vi "WSVCAP SHL Host LL Manage FPGA Top Level Controls.vi"(0 "Value In":variant, 1 "FPGA VI Reference (Init Only)":refnum<k20>, 7 "FPGA Top Level Control":T1=enum."Read Status Flag", 11 "error in (no error)":errorcluster, 12 "Simulate FPGA (Init Only)":bool=TRUE, 13 "Operation":T2) -> (4 "Value Out":variant, 15 "error out":errorcluster)   [LabVIEW 2012]
uses:
  Type Defs/WSVCAP SHL Top Level Control Operation Enum.ctl
  Type Defs/WSVCAP SHL Top Level Control Enum.ctl
  Type Defs/WSVCAP SHL State.ctl
  Type Defs/WSVCAP SHL Transaction Enum.ctl
  <vilib>/Utility/error.llb/Error Cluster From Error Code.vi
  <vilib>/rvi/errors/niLvFpgaAdjustHostInterfaceError.vi
  <vilib>/rvi/interface/nirviReadWriteControl/nirviReadWriteControl.xnode
  FPGA Bitfiles/WSVCAPShell_WiSpryFPGA1_WSVCAPSHLFPGATLT_T3ca54mRgtw.lvbitx
  NiFpgaLv.dll
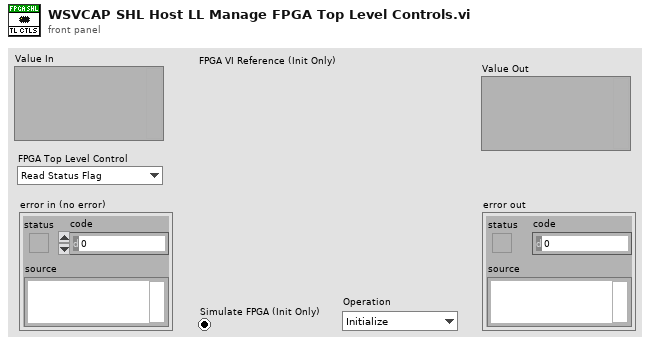
[diagram p1: front panel]
types:
  T1 = typedef "WSVCAP SHL Top Level Control Enum.ctl" = enum16{"Start", "Cmd", "Transaction", "Wait Ticks", "Socket Mask", "Slave Address", "Sub Address", "Bytes to Write", "Bytes to Read", "Write Data", "Write Flag", "Read Data", "Read Flag", "Ack Read", "Read Status Flag", "Ack Read Status", "Status", "Cycle Count", "Stop Cycle", "Exit"}
  T2 = typedef "WSVCAP SHL Top Level Control Operation Enum.ctl" = enum16{"Initialize", "Set Control", "Read Control", "Close"}
  T3 = typedef "WSVCAP SHL State.ctl" = enum8{"Idle", "Transfer Data"}
  T4 = typedef "WSVCAP SHL Transaction Enum.ctl" = enum16{"I2C-Read Data", "I2C-Write Data", "SPI-Write/Read Data", "RFFE-Ext Write", "RFFE-Ext Read"}
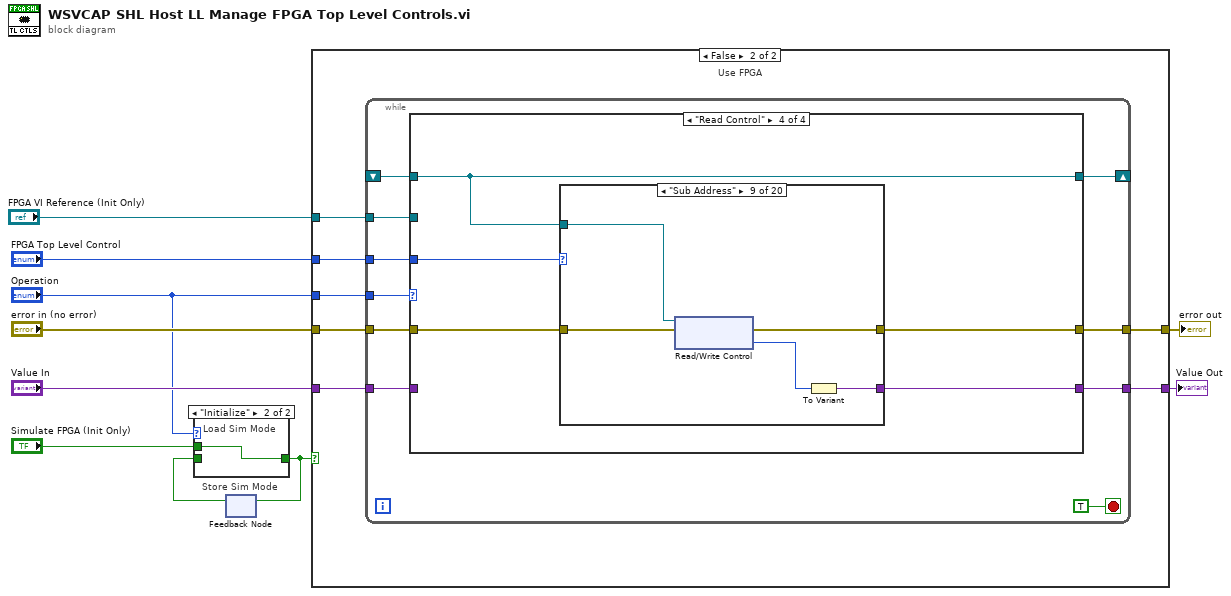
[diagram p0: block diagram]
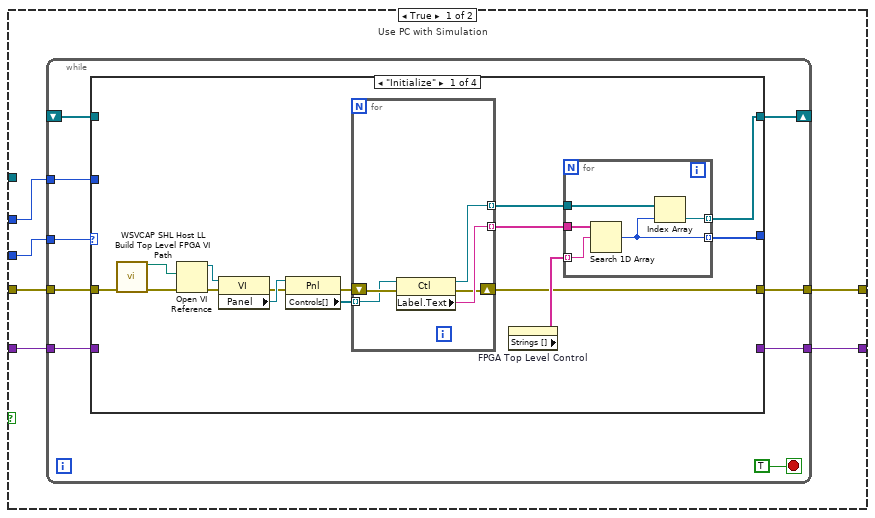
[diagram p2: hidden frame]
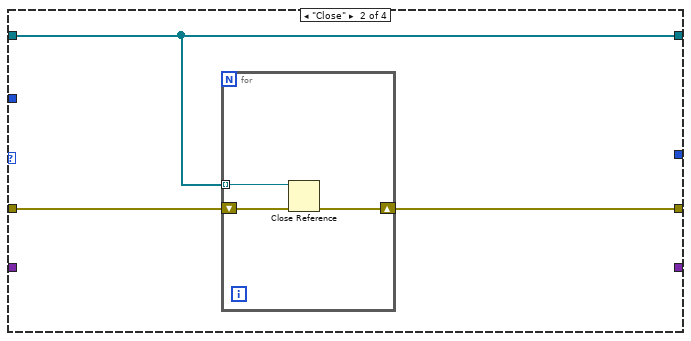
[diagram p3: hidden frame]
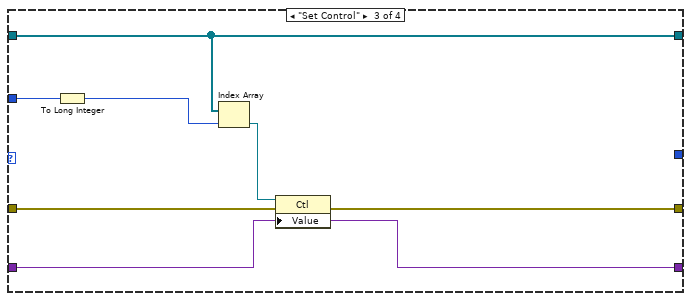
[diagram p4: hidden frame]
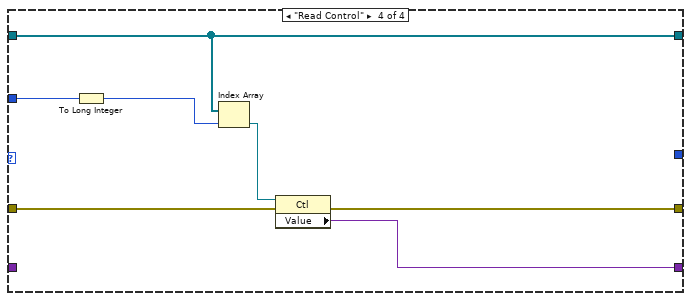
[diagram p5: hidden frame]
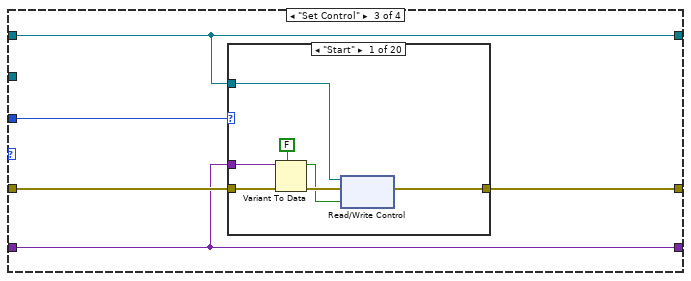
[diagram p8: hidden frame]
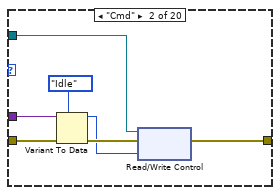
[diagram p9: hidden frame]
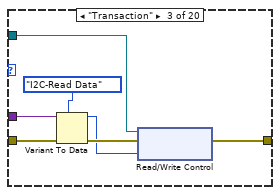
[diagram p10: hidden frame]
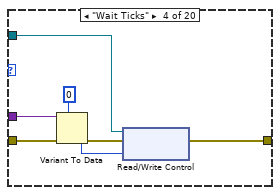
[diagram p11: hidden frame]
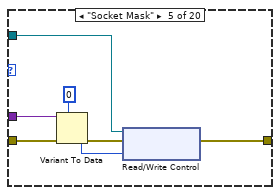
[diagram p12: hidden frame]
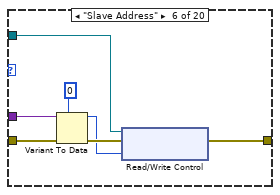
[diagram p13: hidden frame]
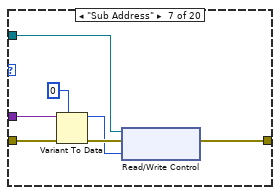
[diagram p14: hidden frame]
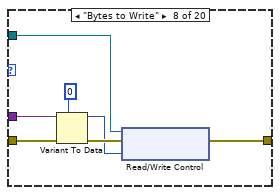
[diagram p15: hidden frame]
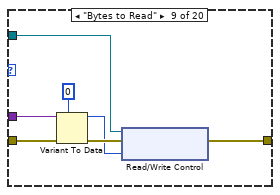
[diagram p16: hidden frame]
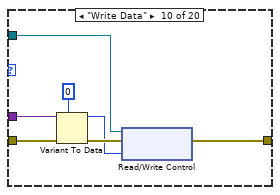
[diagram p17: hidden frame]
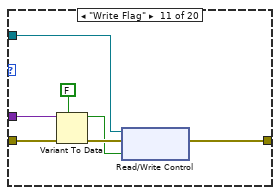
[diagram p18: hidden frame]
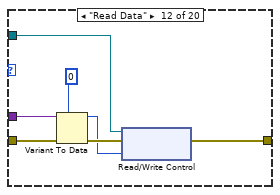
[diagram p19: hidden frame]
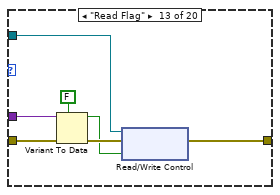
[diagram p20: hidden frame]
diagram:
  # "Store Sim Mode"
  n1 = feedback #1() -> (w2:bool)  [unwired: 1 in]
  n2 = case shown="\"Initialize\"" "Operation" {
    tunnel: [w11 w12] -> w1
    tunnel: "Simulate FPGA (Init Only)" -> [_ w12]
    tunnel: w2 -> [w11 _]
    frame Default {
    }
    frame "Initialize" {
      # "Load Sim Mode"
    }
  }
  n3 = feedback-in #1(w1) -> ()
  n4 = case shown="False" w1 {
    tunnel: "Operation" -> [w18 w79]
    tunnel: [w17 w78] -> w10
    tunnel: "error in (no error)" -> [w16 w77]
    tunnel: [w15 w76] -> w8
    tunnel: "Value In" -> [w14 w75]
    tunnel: "FPGA Top Level Control" -> [w13 w74]
    tunnel: "FPGA VI Reference (Init Only)" -> [_ w73]
    frame True {
      # "Use PC with Simulation"
      n5 = while {
        shift-right: [w27] -> _
        shift-left: _ -> [w25]
        tunnel: w18 -> [w24]
        tunnel: [w23] -> w17
        tunnel: w16 -> [w22]
        tunnel: [w21] -> w15
        tunnel: w14 -> [w20]
        tunnel: w13 -> [w19]
        stop <- TRUE stop-if-true
        n6 = case shown="\"Initialize\"" w24 {
          tunnel: [w36 w55 w65 w72] -> w27
          tunnel: w25 -> [_ w55 w65 w72]
          tunnel: [w32 w54 w62 w69] -> w23
          tunnel: w22 -> [w30 w53 w63 w70]
          tunnel: [_ _ w61 w68] -> w21
          tunnel: w20 -> [_ _ w61 _]
          tunnel: w19 -> [_ _ w60 w67]
          tunnel: [w31 _ _ _] -> _
          frame "Initialize" {
            n7 = call "WSVCAP SHL Host LL Build Top Level FPGA VI Path.vi"("Error In (no error)"=w30) -> ("Top Level FPGA VI Path"=w28:path, "Error Out"=w29:errorcluster)  [unwired: 13 in]
            n8 = Open VI Reference(vi path=w28, error in (no error)=w29) -> (vi reference=w42:refnum<vi>, error out=w35:errorcluster)  [unwired: 4 in]
            n9 = property class="VI"(reference=w42, error in=w35) -> (error out=w34:errorcluster, "Panel"=w41:refnum<vi>)  [unwired: 1 out]
            n10 = property class="Pnl"(reference=w41, error in=w34) -> (error out=w33:errorcluster, "Controls[]"=w40:refnum<vi>[])  [unwired: 1 out]
            n11 = for {
              tunnel: w40 -> [w48] mode=indexing
              tunnel: [w52] -> w37 mode=indexing
              tunnel: [w51] -> w39 mode=indexing
              shift-right: [w49] -> w32
              shift-left: w33 -> [w50]
              n12 = property class="Ctl"(reference=w48, error in=w50) -> (reference out=w52:refnum<vi>, error out=w49:errorcluster, "Label.Text"=w51:string)
            }
            n13 = property on="FPGA Top Level Control" class="Enum (strict)"() -> ("Strings []"=w38:string[])  [unwired: 2 in, 2 out]
            n14 = for {
              tunnel: w39 -> [w47]
              tunnel: w38 -> [w46] mode=indexing
              tunnel: w37 -> [w45]
              tunnel: [w44] -> w36 mode=indexing
              tunnel: [w43] -> w31 mode=indexing
              n15 = Search 1D Array(1D array=w47, element=w46) -> (index of element=w43:i32)  [unwired: 1 in]
              n16 = Index Array(array=w45, index=w43) -> (element=w44:refnum<vi>)
            }
          }
          frame "Close" {
            n17 = for {
              tunnel: w55 -> [w58] mode=indexing
              shift-right: [w57] -> w54
              shift-left: w53 -> [w56]
              n18 = Close Reference(reference=w58, error in (no error)=w56) -> (error out=w57:errorcluster)
            }
          }
          frame "Set Control" {
            n19 = To Long Integer(number=w60) -> (32bit integer=w59:i32)
            n20 = Index Array(array=w65, index=w59) -> (element=w64:refnum<vi>)
            n21 = property class="Ctl"(reference=w64, error in=w63, "Value"=w61) -> (error out=w62:errorcluster)  [unwired: 1 out]
          }
          frame "Read Control" {
            n22 = To Long Integer(number=w67) -> (32bit integer=w66:i32)
            n23 = Index Array(array=w72, index=w66) -> (element=w71:refnum<vi>)
            n24 = property class="Ctl"(reference=w71, error in=w70) -> (error out=w69:errorcluster, "Value"=w68:variant)  [unwired: 1 out]
          }
        }
      }
    }
    frame False {
      # "Use FPGA"
      n25 = while {
        tunnel: w79 -> [w88]
        tunnel: [w87] -> w78
        tunnel: w77 -> [w86]
        tunnel: [w85] -> w76
        tunnel: w75 -> [w84]
        tunnel: w74 -> [w83]
        shift-right: [w82] -> _
        shift-left: _ -> [w81]
        tunnel: w73 -> [w80]
        stop <- TRUE stop-if-true
        n26 = case shown="\"Read Control\"" w88 {
          tunnel: [w90 w93 w97 w241] -> w87
          tunnel: w86 -> [w90 w93 w98 w242]
          tunnel: [_ _ w95 w238] -> w85
          tunnel: w84 -> [_ _ w95 _]
          tunnel: w83 -> [_ _ w96 w240]
          tunnel: [w91 w92 w94 w239] -> w82
          tunnel: w81 -> [_ w92 w94 w239]
          tunnel: w80 -> [w91 _ _ _]
          frame "Initialize" {
          }
          frame "Close" {
          }
          frame "Set Control" {
            n27 = case shown="\"Start\"" w96 {
              tunnel: w94 -> [w105 w112 w119 w126 w133 w140 w147 w154 w161 w168 w175 w182 w189 w196 w203 w210 w217 w223 w230 w237]
              tunnel: w98 -> [w104 w111 w118 w125 w132 w139 w146 w153 w160 w167 w174 w181 w188 w195 w202 w209 w216 w222 w229 w236]
              tunnel: [w102 w109 w116 w123 w130 w137 w144 w151 w158 w165 w172 w179 w186 w193 w200 w207 w214 w220 w227 w234] -> w97
              tunnel: w95 -> [w101 w108 w115 w122 w129 w136 w143 w150 w157 w164 w171 w178 w185 w192 w199 w206 w213 w219 w226 w233]
              frame "Start" {
                n28 = Variant To Data(error in=w104, type=FALSE ("SPI_CPOL"), Variant=w101) -> (data=w100:bool, error out=w103:errorcluster)
                n29 = xnode "Read/Write Control"("FPGA VI Reference In"=w105, "error in"=w103, "Start"=w100) -> ("error out"=w102:errorcluster)  [unwired: 1 out]
              }
              frame "Cmd" {
                n30 = Variant To Data(error in=w111, type=WSVCAP_SHL_State."Idle" ("SPI_Cmd"), Variant=w108) -> (data=w106:T3, error out=w110:errorcluster)
                n31 = xnode "Read/Write Control"("FPGA VI Reference In"=w112, "error in"=w110, "Cmd"=w106) -> ("error out"=w109:errorcluster)  [unwired: 1 out]
              }
              frame "Transaction" {
                n32 = Variant To Data(error in=w118, type=WSVCAP_SHL_Transaction_Enum."I2C-Read Data" ("Transaction"), Variant=w115) -> (data=w113:T4, error out=w117:errorcluster)
                n33 = xnode "Read/Write Control"("FPGA VI Reference In"=w119, "error in"=w117, "Transaction"=w113) -> ("error out"=w116:errorcluster)  [unwired: 1 out]
              }
              frame "Wait Ticks" {
                n34 = Variant To Data(error in=w125, type=u32 0 ("I2C_Clock Divider"), Variant=w122) -> (data=w121:u32, error out=w124:errorcluster)
                n35 = xnode "Read/Write Control"("FPGA VI Reference In"=w126, "error in"=w124, "Wait Ticks"=w121) -> ("error out"=w123:errorcluster)  [unwired: 1 out]
              }
              frame "Socket Mask" {
                n36 = Variant To Data(error in=w132, type=u64 0 ("I2C_Clock Divider"), Variant=w129) -> (data=w128:u64, error out=w131:errorcluster)
                n37 = xnode "Read/Write Control"("FPGA VI Reference In"=w133, "error in"=w131, "Socket Mask"=w128) -> ("error out"=w130:errorcluster)  [unwired: 1 out]
              }
              frame "Slave Address" {
                n38 = Variant To Data(error in=w139, type=u8 0 ("I2C_Slave Address"), Variant=w136) -> (data=w135:u8, error out=w138:errorcluster)
                n39 = xnode "Read/Write Control"("FPGA VI Reference In"=w140, "error in"=w138, "Slave Address"=w135) -> ("error out"=w137:errorcluster)  [unwired: 1 out]
              }
              frame "Sub Address" {
                n40 = Variant To Data(error in=w146, type=u8 0 ("SPI_CS"), Variant=w143) -> (data=w141:u8, error out=w145:errorcluster)
                n41 = xnode "Read/Write Control"("FPGA VI Reference In"=w147, "error in"=w145, "Sub Address"=w141) -> ("error out"=w144:errorcluster)  [unwired: 1 out]
              }
              frame "Bytes to Write" {
                n42 = Variant To Data(error in=w153, type=u8 0 ("SPI_Clock Divider"), Variant=w150) -> (data=w149:u8, error out=w152:errorcluster)
                n43 = xnode "Read/Write Control"("FPGA VI Reference In"=w154, "error in"=w152, "Bytes to Write"=w149) -> ("error out"=w151:errorcluster)  [unwired: 1 out]
              }
              frame "Bytes to Read" {
                n44 = Variant To Data(error in=w160, type=u8 0 ("SPI_Total Bytes"), Variant=w157) -> (data=w156:u8, error out=w159:errorcluster)
                n45 = xnode "Read/Write Control"("FPGA VI Reference In"=w161, "error in"=w159, "Bytes to Read"=w156) -> ("error out"=w158:errorcluster)  [unwired: 1 out]
              }
              frame "Write Data" {
                n46 = Variant To Data(error in=w167, type=u64 0 ("SPI_Total Bytes"), Variant=w164) -> (data=w163:u64, error out=w166:errorcluster)
                n47 = xnode "Read/Write Control"("FPGA VI Reference In"=w168, "error in"=w166, "Write Data"=w163) -> ("error out"=w165:errorcluster)  [unwired: 1 out]
              }
              frame "Write Flag" {
                n48 = Variant To Data(error in=w174, type=FALSE, Variant=w171) -> (data=w170:bool, error out=w173:errorcluster)
                n49 = xnode "Read/Write Control"("FPGA VI Reference In"=w175, "error in"=w173, "Write Flag"=w170) -> ("error out"=w172:errorcluster)  [unwired: 1 out]
              }
              frame "Read Data" {
                n50 = Variant To Data(error in=w181, type=u64 0 ("I2C_Read Data"), Variant=w178) -> (data=w176:u64, error out=w180:errorcluster)
                n51 = xnode "Read/Write Control"("FPGA VI Reference In"=w182, "error in"=w180, "Read Data"=w176) -> ("error out"=w179:errorcluster)  [unwired: 1 out]
              }
              frame "Read Flag" {
                n52 = Variant To Data(error in=w188, type=FALSE ("SPI_CPOL"), Variant=w185) -> (data=w183:bool, error out=w187:errorcluster)
                n53 = xnode "Read/Write Control"("FPGA VI Reference In"=w189, "error in"=w187, "Read Flag"=w183) -> ("error out"=w186:errorcluster)  [unwired: 1 out]
              }
              frame "Ack Read" {
                n54 = Variant To Data(error in=w195, type=FALSE ("SPI_CPOL"), Variant=w192) -> (data=w191:bool, error out=w194:errorcluster)
                n55 = xnode "Read/Write Control"("FPGA VI Reference In"=w196, "error in"=w194, "Ack Read"=w191) -> ("error out"=w193:errorcluster)  [unwired: 1 out]
              }
              frame "Read Status Flag" {
                n56 = Variant To Data(error in=w202, type=FALSE ("SPI_CPOL"), Variant=w199) -> (data=w198:bool, error out=w201:errorcluster)
                n57 = xnode "Read/Write Control"("FPGA VI Reference In"=w203, "error in"=w201, "Read Status Flag"=w198) -> ("error out"=w200:errorcluster)  [unwired: 1 out]
              }
              frame "Ack Read Status" {
                n58 = Variant To Data(error in=w209, type=FALSE ("SPI_CPOL"), Variant=w206) -> (data=w205:bool, error out=w208:errorcluster)
                n59 = xnode "Read/Write Control"("FPGA VI Reference In"=w210, "error in"=w208, "Ack Read Status"=w205) -> ("error out"=w207:errorcluster)  [unwired: 1 out]
              }
              frame "Status" {
                n60 = Variant To Data(error in=w216, type=0 ("I2C_Status"), Variant=w213) -> (data=w211:i32, error out=w215:errorcluster)
                n61 = xnode "Read/Write Control"("FPGA VI Reference In"=w217, "error in"=w215, "Status"=w211) -> ("error out"=w214:errorcluster)  [unwired: 1 out]
              }
              frame "Cycle Count" {
                w218 = u64 0 ("Cycle Count")
                n62 = Variant To Data(error in=w222, type=w218, Variant=w219) -> (error out=w221:errorcluster)  [unwired: 1 out]
                n63 = xnode "Read/Write Control"("FPGA VI Reference In"=w223, "error in"=w221, "Cycle Count"=w218) -> ("error out"=w220:errorcluster)  [unwired: 1 out]
              }
              frame "Stop Cycle" {
                n64 = Variant To Data(error in=w229, type=FALSE ("SPI_CPOL"), Variant=w226) -> (data=w225:bool, error out=w228:errorcluster)
                n65 = xnode "Read/Write Control"("FPGA VI Reference In"=w230, "error in"=w228, "Stop Cycle"=w225) -> ("error out"=w227:errorcluster)  [unwired: 1 out]
              }
              frame "Exit" {
                n66 = Variant To Data(error in=w236, type=FALSE ("I2C_Exit"), Variant=w233) -> (data=w232:bool, error out=w235:errorcluster)
                n67 = xnode "Read/Write Control"("FPGA VI Reference In"=w237, "error in"=w235, "Exit"=w232) -> ("error out"=w234:errorcluster)  [unwired: 1 out]
              }
            }
          }
          frame "Read Control" {
            n68 = case shown="\"Sub Address\"" w240 {
              tunnel: w239 -> [w247 w252 w257 w262 w267 w272 w277 w282 w287 w292 w297 w302 w307 w312 w317 w322 w327 w332 w337 w342]
              tunnel: w242 -> [w245 w250 w255 w258 w263 w268 w273 w280 w285 w289 w295 w300 w305 w310 w315 w320 w325 w330 w335 w340]
              tunnel: [w246 w251 w256 w261 w266 w271 w276 w281 w286 w291 w296 w301 w306 w311 w316 w321 w326 w331 w336 w341] -> w241
              tunnel: [w243 w248 w254 w259 w264 w269 w274 w278 w283 w288 w293 w298 w303 w308 w313 w318 w323 w328 w333 w338] -> w238
              frame "Start" {
                n69 = xnode "Read/Write Control"("FPGA VI Reference In"=w247, "error in"=w245) -> ("error out"=w246:errorcluster, "Start"=w244:bool)  [unwired: 1 out]
                n70 = To Variant(anything=w244) -> (Variant=w243:variant)
              }
              frame "Cmd" {
                n71 = xnode "Read/Write Control"("FPGA VI Reference In"=w252, "error in"=w250) -> ("error out"=w251:errorcluster, "Cmd"=w249:T3)  [unwired: 1 out]
                n72 = To Variant(anything=w249) -> (Variant=w248:variant)
              }
              frame "Transaction" {
                n73 = xnode "Read/Write Control"("FPGA VI Reference In"=w257, "error in"=w255) -> ("error out"=w256:errorcluster, "Transaction"=w253:T4)  [unwired: 1 out]
                n74 = To Variant(anything=w253) -> (Variant=w254:variant)
              }
              frame "Wait Ticks" {
                n75 = xnode "Read/Write Control"("FPGA VI Reference In"=w262, "error in"=w258) -> ("error out"=w261:errorcluster, "Wait Ticks"=w260:u32)  [unwired: 1 out]
                n76 = To Variant(anything=w260) -> (Variant=w259:variant)
              }
              frame "Socket Mask" {
                n77 = xnode "Read/Write Control"("FPGA VI Reference In"=w267, "error in"=w263) -> ("error out"=w266:errorcluster, "Socket Mask"=w265:u64)  [unwired: 1 out]
                n78 = To Variant(anything=w265) -> (Variant=w264:variant)
              }
              frame "Cycle Count" {
                n79 = xnode "Read/Write Control"("FPGA VI Reference In"=w272, "error in"=w268) -> ("error out"=w271:errorcluster, "Cycle Count"=w270:u64)  [unwired: 1 out]
                n80 = To Variant(anything=w270) -> (Variant=w269:variant)
              }
              frame "Stop Cycle" {
                n81 = xnode "Read/Write Control"("FPGA VI Reference In"=w277, "error in"=w273) -> ("error out"=w276:errorcluster, "Stop Cycle"=w275:bool)  [unwired: 1 out]
                n82 = To Variant(anything=w275) -> (Variant=w274:variant)
              }
              frame "Slave Address" {
                n83 = xnode "Read/Write Control"("FPGA VI Reference In"=w282, "error in"=w280) -> ("error out"=w281:errorcluster, "Slave Address"=w279:u8)  [unwired: 1 out]
                n84 = To Variant(anything=w279) -> (Variant=w278:variant)
              }
              frame "Sub Address" {
                n85 = xnode "Read/Write Control"("FPGA VI Reference In"=w287, "error in"=w285) -> ("error out"=w286:errorcluster, "Sub Address"=w284:u8)  [unwired: 1 out]
                n86 = To Variant(anything=w284) -> (Variant=w283:variant)
              }
              frame "Bytes to Write" {
                n87 = xnode "Read/Write Control"("FPGA VI Reference In"=w292, "error in"=w289) -> ("error out"=w291:errorcluster, "Bytes to Write"=w290:u8)  [unwired: 1 out]
                n88 = To Variant(anything=w290) -> (Variant=w288:variant)
              }
              frame "Bytes to Read" {
                n89 = xnode "Read/Write Control"("FPGA VI Reference In"=w297, "error in"=w295) -> ("error out"=w296:errorcluster, "Bytes to Read"=w294:u8)  [unwired: 1 out]
                n90 = To Variant(anything=w294) -> (Variant=w293:variant)
              }
              frame "Write Data" {
                n91 = xnode "Read/Write Control"("FPGA VI Reference In"=w302, "error in"=w300) -> ("error out"=w301:errorcluster, "Write Data"=w299:u64)  [unwired: 1 out]
                n92 = To Variant(anything=w299) -> (Variant=w298:variant)
              }
              frame "Write Flag" {
                n93 = xnode "Read/Write Control"("FPGA VI Reference In"=w307, "error in"=w305) -> ("error out"=w306:errorcluster, "Write Flag"=w304:bool)  [unwired: 1 out]
                n94 = To Variant(anything=w304) -> (Variant=w303:variant)
              }
              frame "Read Data" {
                n95 = xnode "Read/Write Control"("FPGA VI Reference In"=w312, "error in"=w310) -> ("error out"=w311:errorcluster, "Read Data"=w309:u64)  [unwired: 1 out]
                n96 = To Variant(anything=w309) -> (Variant=w308:variant)
              }
              frame "Read Flag" {
                n97 = xnode "Read/Write Control"("FPGA VI Reference In"=w317, "error in"=w315) -> ("error out"=w316:errorcluster, "Read Flag"=w314:bool)  [unwired: 1 out]
                n98 = To Variant(anything=w314) -> (Variant=w313:variant)
              }
              frame "Ack Read" {
                n99 = xnode "Read/Write Control"("FPGA VI Reference In"=w322, "error in"=w320) -> ("error out"=w321:errorcluster, "Ack Read"=w319:bool)  [unwired: 1 out]
                n100 = To Variant(anything=w319) -> (Variant=w318:variant)
              }
              frame "Read Status Flag" {
                n101 = xnode "Read/Write Control"("FPGA VI Reference In"=w327, "error in"=w325) -> ("error out"=w326:errorcluster, "Read Status Flag"=w324:bool)  [unwired: 1 out]
                n102 = To Variant(anything=w324) -> (Variant=w323:variant)
              }
              frame "Ack Read Status" {
                n103 = xnode "Read/Write Control"("FPGA VI Reference In"=w332, "error in"=w330) -> ("error out"=w331:errorcluster, "Ack Read Status"=w329:bool)  [unwired: 1 out]
                n104 = To Variant(anything=w329) -> (Variant=w328:variant)
              }
              frame "Status" {
                n105 = xnode "Read/Write Control"("FPGA VI Reference In"=w337, "error in"=w335) -> ("error out"=w336:errorcluster, "Status"=w334:i32)  [unwired: 1 out]
                n106 = To Variant(anything=w334) -> (Variant=w333:variant)
              }
              frame "Exit" {
                n107 = xnode "Read/Write Control"("FPGA VI Reference In"=w342, "error in"=w340) -> ("error out"=w341:errorcluster, "Exit"=w339:bool)  [unwired: 1 out]
                n108 = To Variant(anything=w339) -> (Variant=w338:variant)
              }
            }
          }
        }
      }
    }
  }
  "error out" <- w10
  "Value Out" <- w8
